vi "save_to_file.vi"   [LabVIEW 2016]
uses:
  <vilib>/Utility/file.llb/Write Delimited Spreadsheet (DBL).vi
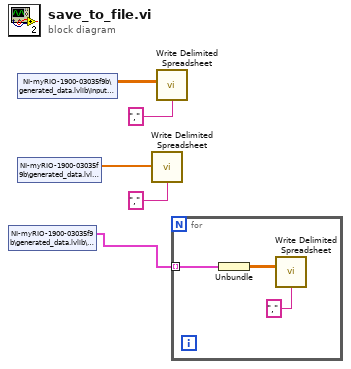
[diagram p0: block diagram]
diagram:
  n1 = shared-variable "NI-myRIO-1900-03035f9b\\generated_data.lvlib\\Weights"() -> (w1:cluster{dbl[][]}[])  [unwired: 1 in, 1 out]
  n2 = shared-variable "NI-myRIO-1900-03035f9b\\generated_data.lvlib\\Input Data"() -> (w5:dbl[][])  [unwired: 1 in, 1 out]
  n3 = shared-variable "NI-myRIO-1900-03035f9b\\generated_data.lvlib\\Targets"() -> (w3:dbl[])  [unwired: 1 in, 1 out]
  n4 = call-poly <vilib>:"Write Delimited Spreadsheet.vi"("1D data"=w3, "delimiter (\\t)"=",") -> ()  [unwired: 12 in, 2 out]
  n5 = call-poly <vilib>:"Write Delimited Spreadsheet.vi"("2D data"=w5, "delimiter (\\t)"=",") -> ()  [unwired: 12 in, 2 out]
  n6 = for {
    tunnel: w1 -> [w8] mode=indexing
    n7 = Unbundle(w8) -> (w7:dbl[][])
    n8 = call-poly <vilib>:"Write Delimited Spreadsheet.vi"("2D data"=w7, "delimiter (\\t)"=",") -> ()  [unwired: 12 in, 2 out]
  }
